vi "Insert Error.vi"(8 "error in":errorcluster, 10 "err":errorcluster, 11 "Instrument in":refnum<class "Instrument.lvclass">) -> (0 "error out":errorcluster, 2 "error?":bool, 3 "Instrument out":refnum<class "Instrument.lvclass">)   [LabVIEW 2016, in "Instrument.lvclass"]
doc: "Insert an error into the error queue in the Instrument class. If the queue has been recently cleared (as indicated by the Error to Handle? flag set to false, then set this flag so that errors may be properly handled."
uses:
  Instrument.lvclass
  Instrument.lvclass/Instrument.ctl
  state.ctl
  Session APIs/Session Log/System Log.lvclass
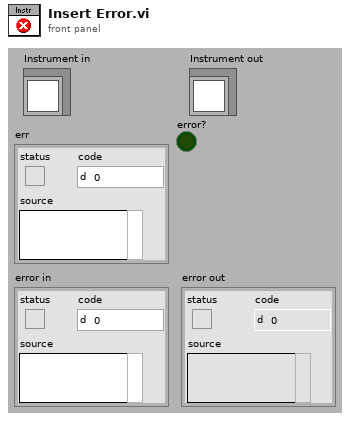
[diagram p1: front panel]
types:
  T1 = typedef "Instrument.lvclass/state.ctl" = enum8{"Configure", "Acquire", "Wait", "Quit", "Handle Error", "NOOP"}
  T2 = typedef "Session - Root.lvclass/Session Handle.ctl" = refnum<data-value>
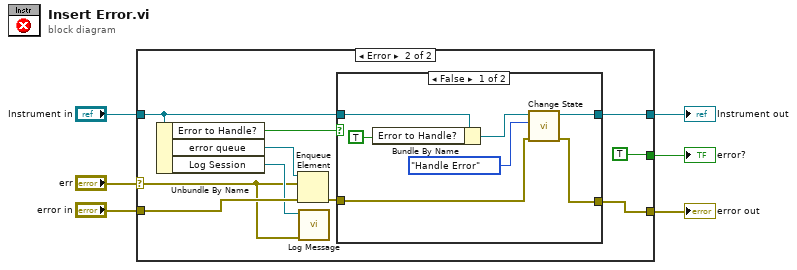
[diagram p0: block diagram]
diagram:
  n1 = case shown="Error" "err" {
    selector: "err" -> [_ w9]
    tunnel: "Instrument in" -> [w7 w15]
    tunnel: "error in" -> [w8 w17]
    tunnel: [w8 w12] -> w5
    tunnel: [_ TRUE] -> w1
    tunnel: [w7 w11] -> w3
    frame No Error {
    }
    frame Error {
      n2 = Unbundle By Name(w15) -> ("Error to Handle?"=w14:bool, "error queue"=w18:refnum<queue>, "Log Session"=w10:T2)
      n3 = Enqueue Element(queue=w18, element=w9, error in (no error)=w17) -> (error out=w13:errorcluster)  [unwired: 1 in, 2 out]
      n4 = call "Log Message.vi"("error in"=w9, "session in"=w10) -> ()  [unwired: 8 in, 2 out]
      n5 = case shown="False" w14 {
        tunnel: w15 -> [w24 w26]
        tunnel: [w22 w26] -> w11
        tunnel: w13 -> [w20 w27]
        tunnel: [w19 w27] -> w12
        frame False {
          n6 = Bundle By Name(cluster=w24, "Error to Handle?"=TRUE) -> (w23:refnum<class "Instrument.lvclass">)
          n7 = call "Change State.vi"("error in"=w20, "instr state"=state."Handle Error", "Instrument in"=w23) -> ("error out"=w19:errorcluster, "Instrument out"=w22:refnum<class "Instrument.lvclass">)  [unwired: 7 in]
        }
        frame True {
        }
      }
    }
  }
  "error out" <- w5
  "Instrument out" <- w3
  "error?" <- w1
